vi "Eagle Scanner and Illumination Control V1.vi"() -> ()   [LabVIEW 2015]
uses:
  <vilib>/userdefined/High Color/IMAQdx.ctl
  <vilib>/vision/Image Controls.llb/IMAQ Image.ctl
  IP Dev Area/IP results.ctl
  <vilib>/FPGAPlugInAG/cRIO-9030/niLvFpga_Open_cRIO-9030.vi
  <vilib>/rvi/interface/common/dynamic/niFpgaDynamicAddResources.vi
  <vilib>/FPGAPlugInAG/Dynamic/niLvFpga_Download_Dynamic.vi
  <vilib>/FPGAPlugInAG/Dynamic/niLvFpga_Run_Dynamic.vi
  <vilib>/Utility/error.llb/Error Cluster From Error Code.vi
  <vilib>/rvi/errors/niLvFpgaAdjustHostInterfaceError.vi
  <vilib>/rvi/interface/nirviOpenFPGA/nirviOpenFPGA.xnode
  FPGA Bitfiles/BELKINEAGLEGUI_FPGATarget_EagleFPGAScanner_lK+EHUuZRCQ.lvbitx
  <vilib>/rvi/interface/nirviMethod/nirviMethod.xnode
  <vilib>/rvi/interface/nirviReadWriteControl/nirviReadWriteControl.xnode
  <vilib>/rvi/interface/Simulation/niFpgaSimulationCallBeginRW.vi
  NiFpgaLv.dll
  <vilib>/Utility/miscctls.llb/LVRectTypeDef.ctl
  <vilib>/vision/driver/NI_Vision_Acquisition_Software.lvlib
  <vilib>/vision/NI_Vision_Development_Module.lvlib
panel:
  out "LiveImageBuffer":T1
  in  "LiveVideo":bool
  out "ImagesFolder":path
  out "ImageBuffer":T1
  out "IMAQ Session":T2 caption="Session Out"
  in  "Auto Scanner":bool
  out "Tab Control":T3(tab)
  in  "Images Root Folder":path
  in  "LED Ctrl":dbl(slide)=1.0 caption="LED Ring" max=100.0 step=1.0 scale=0.0..100.0 scale format="%#.3g"
  in  "Red Dots Ctrl":dbl(slide)=1.0 caption="Red Dots" max=100.0 step=1.0 scale=0.0..100.0 scale format="%#.3g"
  in  "Number Of Points AC":u16=100 caption="Number Of Points"
  in  "Dwell Time":dbl=1.0 caption="Dwell Time [Sec]"
  in  "Radius A AC":dbl caption="Radius A [Volt]"
  in  "Radius B AC":dbl caption="Radius B [Volt]"
  in  "VY OFFS [Volt] AC":fxp<+/-,20,5> caption="VY OFFS [Volt]"
  in  "VX OFFS [Volt] AC":fxp<+/-,20,5> caption="VX OFFS [Volt]"
  out "Image":T1(plugin-control)
  in  "Run":bool
  in  "Stop":bool
  in  "A ON":bool caption="On/Off"
  in  "H ON":bool caption="On/Off"
  in  "V ON":bool caption="On/Off"
  in  "Aiming Ctrl":dbl=1.0 caption="Aiming" max=100.0 step=1.0
  in  "H Range Ctrl":dbl=1.0 caption="H Range" max=100.0 step=1.0
  in  "V Range Ctrl":dbl=1.0 caption="V Range" max=100.0 step=1.0
  in  "Scanner X":dbl=6.712328767123287 caption="X Control" min=-10.0 max=10.0 step=1.0
  in  "Scanner Y":dbl=1.5068493150684925 caption="Y Control" min=-10.0 max=10.0 step=1.0
  out "X IND":fxp<+/-,20,5>
  out "Y IND":fxp<+/-,20,5>
  in  "Send":bool
  out "X Readback Man":fxp<+/-,20,5> caption="X Readback [Volt]"
  out "Y Readback Man":fxp<+/-,20,5> caption="Y Readback [Volt]"
  out "Sensor 1":dbl
  out "Sensor 2":dbl
  out "Live Image":T1(plugin-control)
  in  "Grab":bool
  out "X Graph":u16[](graph) caption="Brightness Distribution [X]"
  out "Y Graph":u16[](graph) caption="Brightness Distribution [Y]"
  in  "AutoPlot":bool caption="Mark this to show distribution\nof the brightest point"
  in  "Snap":bool
  in  "Save":bool
  out "Y Readback":fxp<+/-,20,5> caption="Y Readback [Volt]"
  out "X Readback":fxp<+/-,20,5> caption="X Readback [Volt]"
  out "Y Command":fxp<+/-,20,5> caption="Y Command [Volt]"
  out "X Command":fxp<+/-,20,5> caption="X Command [Volt}"
  in  "Radius B":dbl caption="Radius B [Volt]"
  in  "Radius A":dbl caption="Radius A [Volt]"
  in  "Velocity":dbl=1.0 caption="Velocity [R/Sec]"
  in  "Number Of Points":u16=100
  in  "FreeRun":bool
  in  "VX OFFS [Volt]":fxp<+/-,20,5>
  in  "VY OFFS [Volt]":fxp<+/-,20,5>
  in  "Scanner FreeRun":bool
  in  "Manual Scanner":bool
  out "Stopped":bool
  in  "stop":bool
  # "EAGLE SYSTEM BASIC CONTROL"
  # "Automatic Scanner Control"
  # "Live Video"
  # "Manual Control"
  # "Illumination Control"
  # "Camera Control"
  # "Scanner Control"
  # "Otherwise touch the image at the point of interest"
  # "Temperature Sensors"
  # "Scanner Free Run"
  # "General Parameters"
  # "Calibration Parameters"
  # "Position Indication"
  # "Trajectory Parameters"
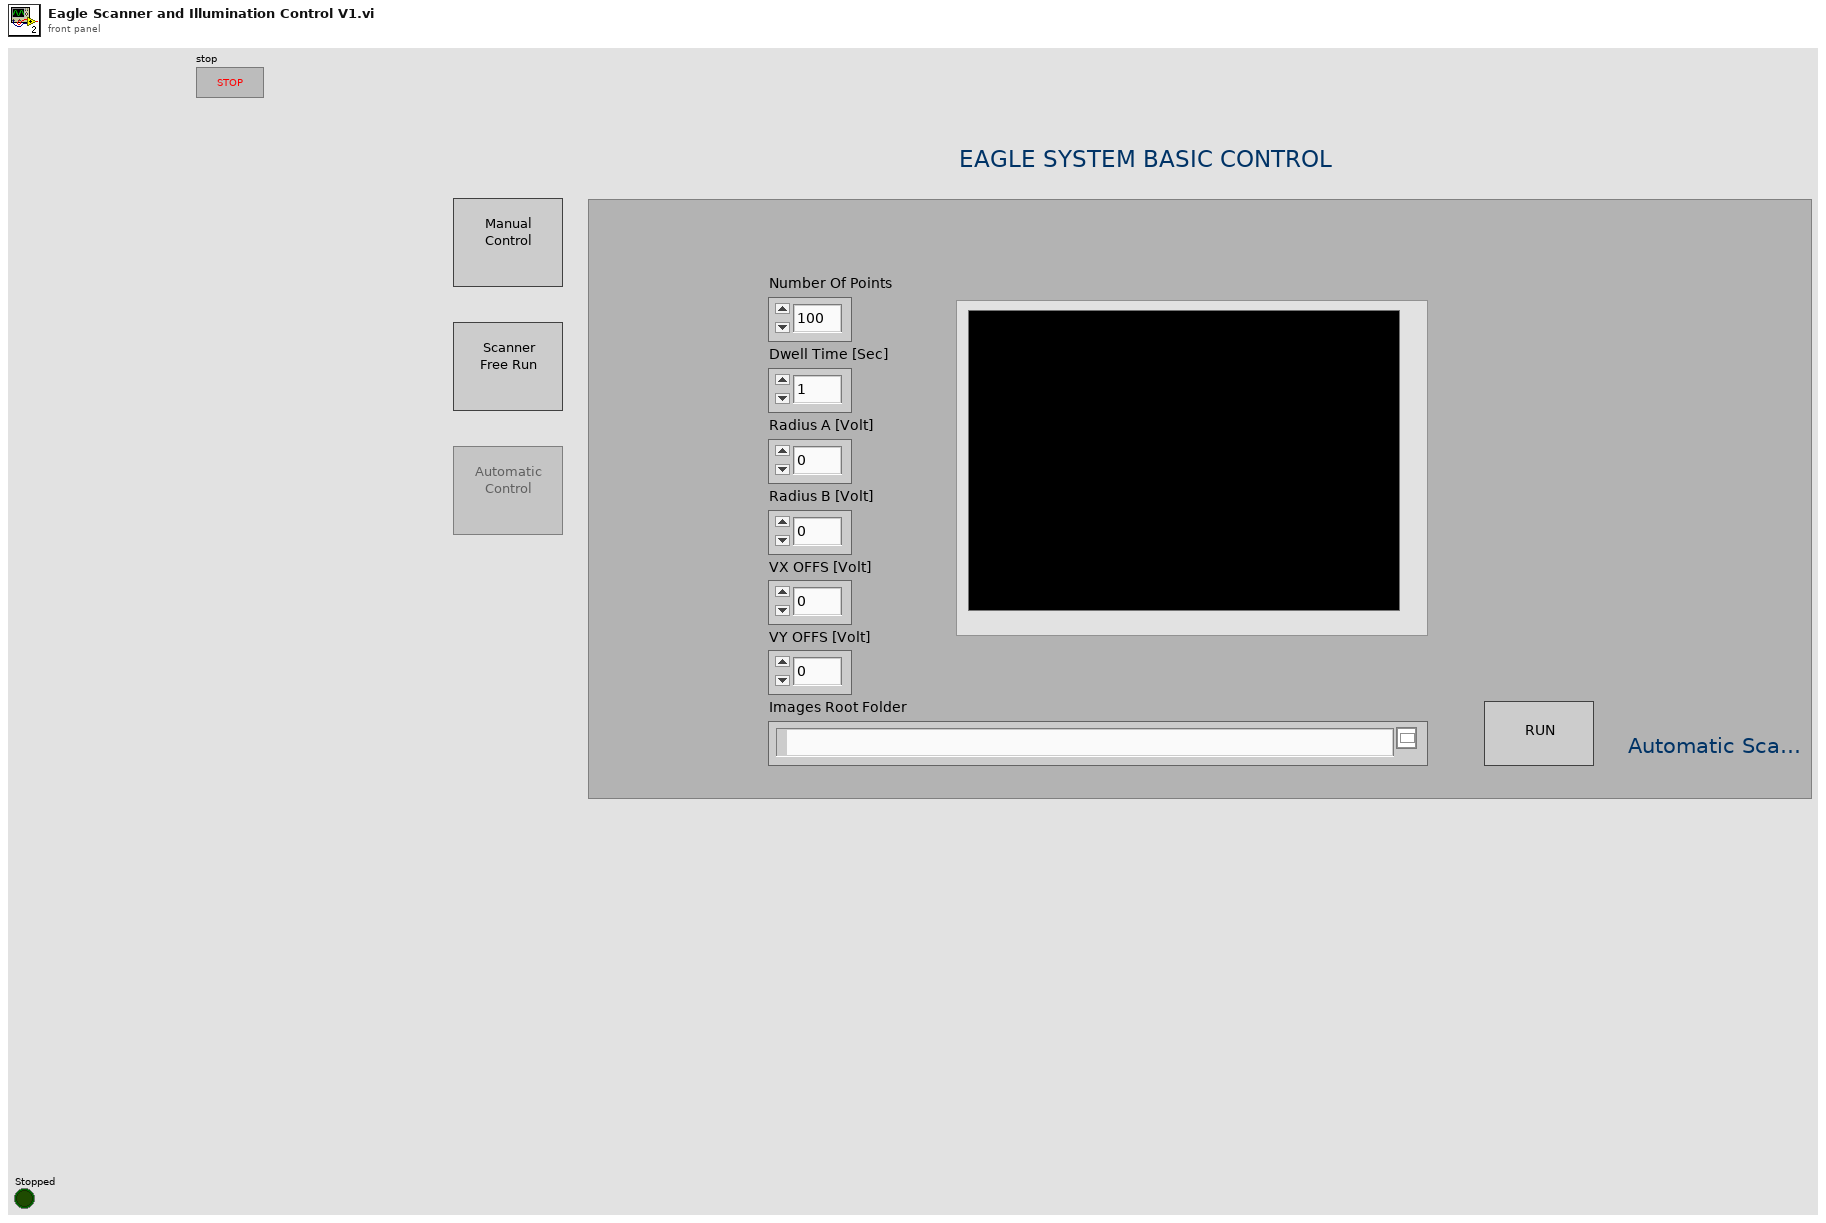
[diagram p1: front panel]
types:
  T1 = typedef "IMAQ Image.ctl" = refnum<image>
  T2 = typedef "IMAQdx.ctl" = refnum<k21>
  T3 = enum32{"Automatic", "Video Live", "Manual", "Free Run"}
  T4 = typedef "LVRectTypeDef.ctl" = cluster{"Left":i16, "Top":i16, "Right":i16, "Bottom":i16}
  T5 = cluster{"LedRing_Ctrl":dbl, "RedDots_Ctrl":dbl, "VRange_Ctrl":dbl, "HRange_Ctrl":dbl, "Aim_Ctrl":dbl, "ScanX":dbl, "ScanY":dbl, "Trajectory":cluster{"Radius A":dbl, "Radius B":dbl, "VX OFFS":fxp<+/-,20,5>, "VY OFFS":fxp<+/-,20,5>}, "General":cluster{"NumOfPoints":u16, "Velocity":dbl}, "Tab":u32, "Automatic":cluster{"NumOfPoints":u16, "Dwell Time":dbl, "VY OFFS":fxp<+/-,20,5>, "VX OFFS":fxp<+/-,20,5>, "Radius A":dbl, "Radius B":dbl}, "Images Folder":path}
  T6 = typedef "IP results.ctl" = cluster{"X":u16, "Y":u16, "A":dbl, "B":dbl, "Grade":u16, "Frame#":u16}
  T7 = enum8{"Enabled", "Disabled", "Disabled and Grayed Out"}
  T8 = typedef "Image Type" = u32
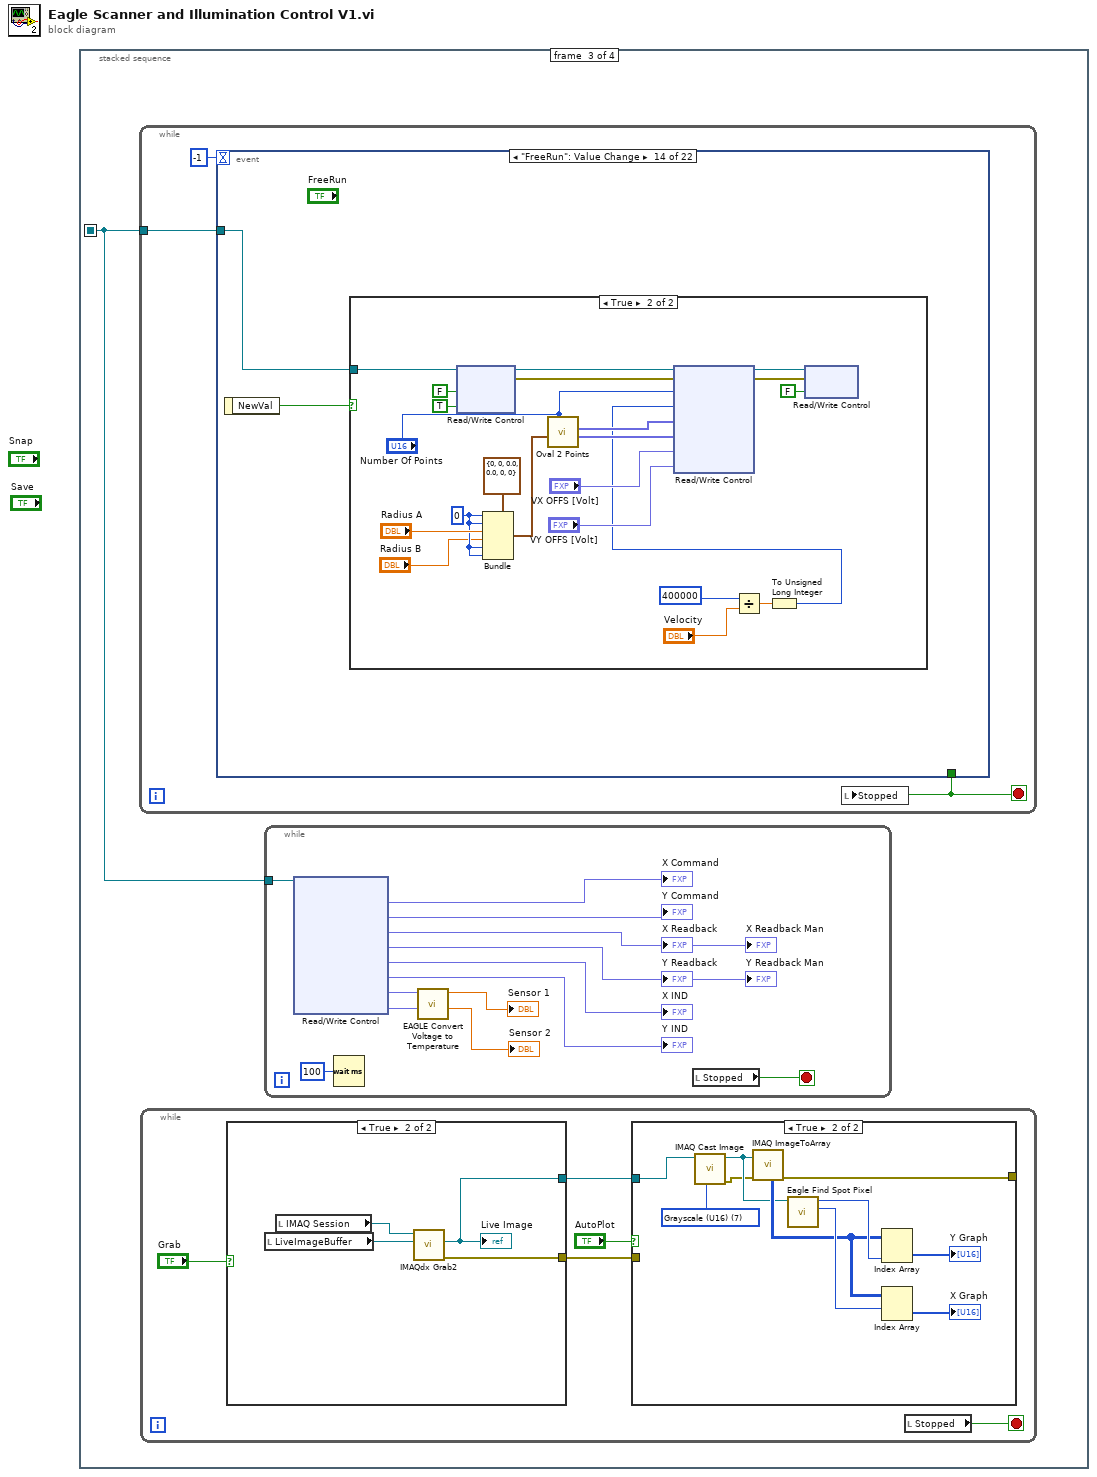
[diagram p0: block diagram]
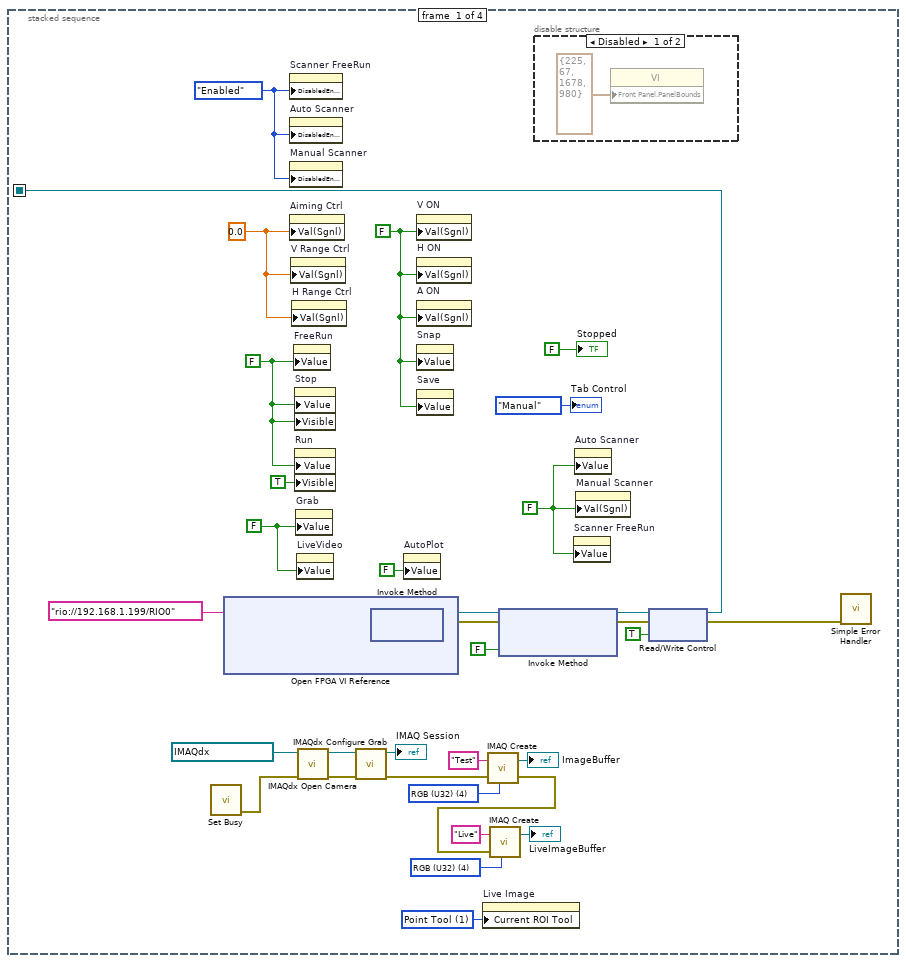
[diagram p2: hidden frame]
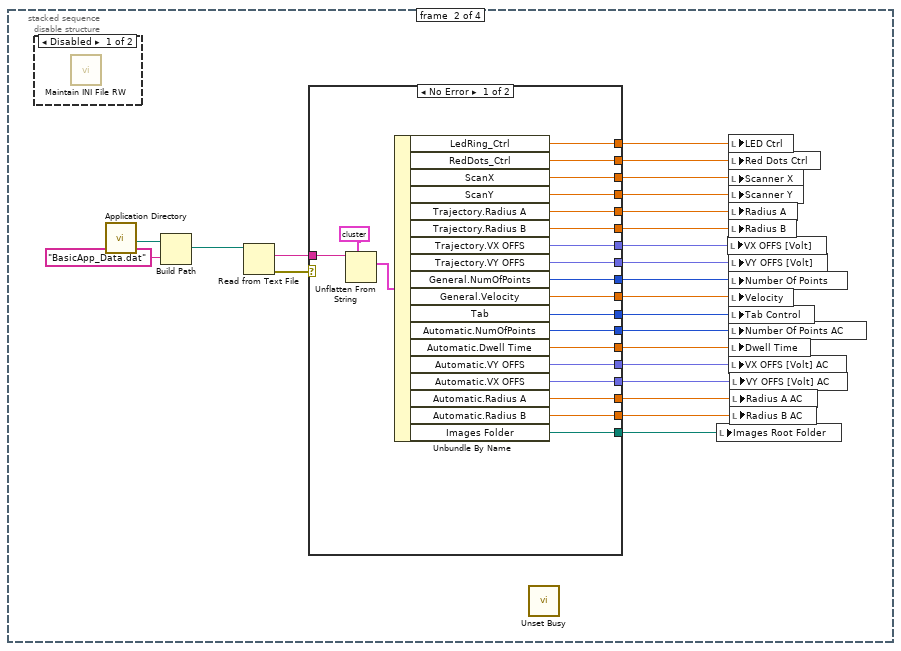
[diagram p4: hidden frame]
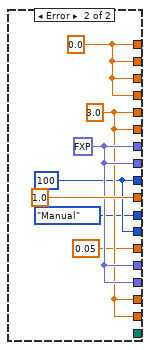
[diagram p6: hidden frame]
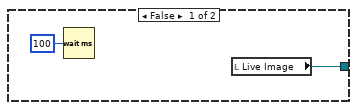
[diagram p8: hidden frame]
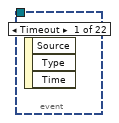
[diagram p9: hidden frame]
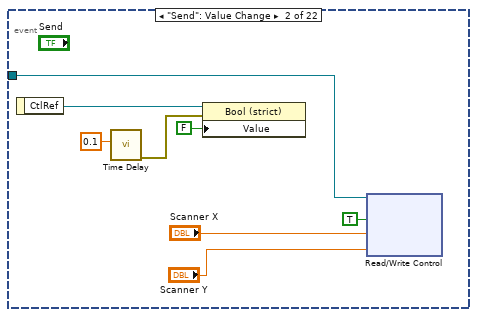
[diagram p10: hidden frame]
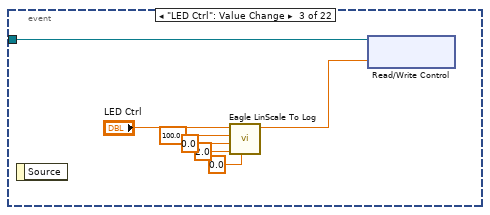
[diagram p11: hidden frame]
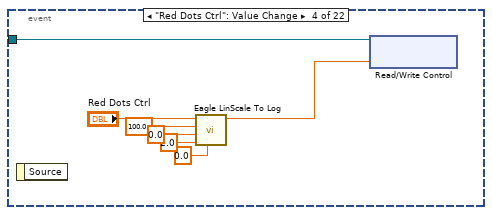
[diagram p12: hidden frame]
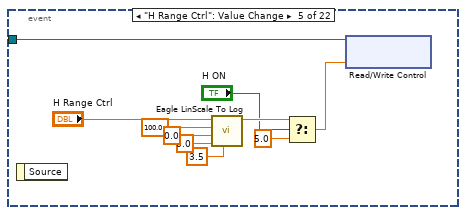
[diagram p13: hidden frame]
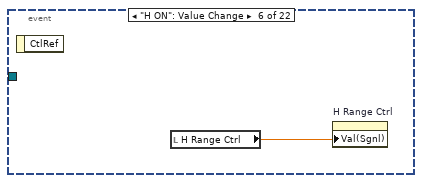
[diagram p14: hidden frame]
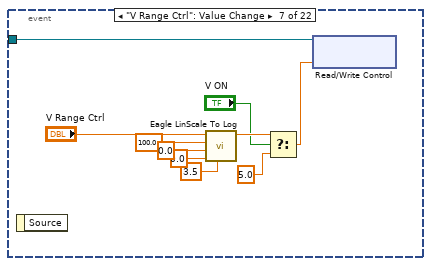
[diagram p15: hidden frame]
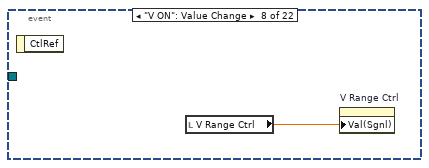
[diagram p16: hidden frame]
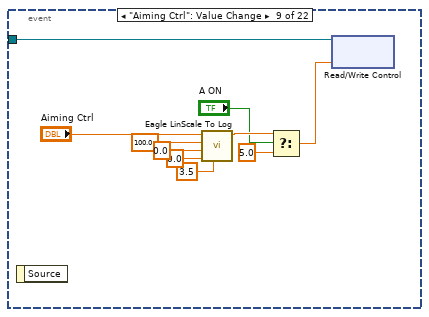
[diagram p17: hidden frame]
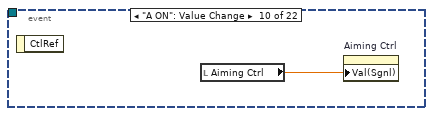
[diagram p18: hidden frame]
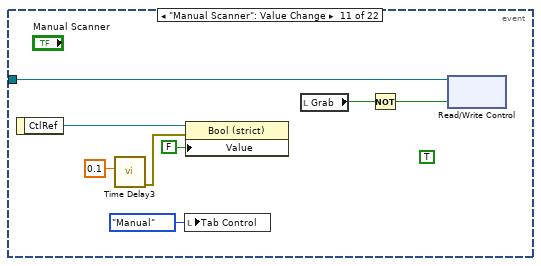
[diagram p19: hidden frame]
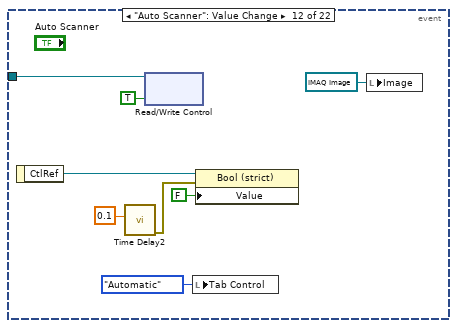
[diagram p20: hidden frame]
diagram:
  n1 = stacked-sequence {
    seq-local: [w33 _ _ _] -> [_ _ w88 _]
    frame #0 {
      w1 = FALSE
      w2 = u32 1 items=["Zoom Tool"=8, "Selection Tool"=0, "Pan Tool"=9, "Point Tool"=1, "Line Tool"=2, "Rectangle Tool"=3, "Rotated Rectangle Tool"=12, "Polyline Tool"=10, "Polygon Tool"=5, "Freehand Tool"=11, "Closed Freehand Tool"=6, "Ellipse Tool"=4, "Annulus Tool"=7] ("Current ROI Tool")
      w5 = T8 4 items=["Grayscale (U8)", "Grayscale (I16)", "Grayscale (SGL)", "Complex (CSG)", "RGB (U32)", "HSL (U32)", "RGB (U64)", "Grayscale (U16)"] ("Image Type")
      w8 = T8 4 items=["Grayscale (U8)", "Grayscale (I16)", "Grayscale (SGL)", "Complex (CSG)", "RGB (U32)", "HSL (U32)", "RGB (U64)", "Grayscale (U16)"] ("Image Type")
      w18 = FALSE ("Start Live")
      w20 = T7."Enabled" ("Disabled")
      w22 = FALSE ("FreeRun")
      w24 = 0.0 ("Value (Signaling)")
      w23 = FALSE
      n2 = call <vilib>:"Set Busy.vi"() -> ("error out"=w6:errorcluster)  [unwired: 10 in, 1 out]
      n3 = xnode "Open FPGA VI Reference"("resource name"=tag "rio://192.168.1.199/RIO0") -> ("FPGA VI Reference Out"=w30:refnum<k20>, "error out"=w29:errorcluster)  [unwired: 1 in]
      n4 = property on="Scanner FreeRun" class="Bool (strict)"("DisabledEnum"=w20) -> ()  [unwired: 2 in, 2 out]
      n5 = property on="Auto Scanner" class="Bool (strict)"("DisabledEnum"=w20) -> ()  [unwired: 2 in, 2 out]
      n6 = property on="Manual Scanner" class="Bool (strict)"("DisabledEnum"=w20) -> ()  [unwired: 2 in, 2 out]
      n7 = property on="Aiming Ctrl" class="DigNum (strict)"("Val(Sgnl)"=w24) -> ()  [unwired: 2 in, 2 out]
      n8 = property on="V Range Ctrl" class="DigNum (strict)"("Val(Sgnl)"=w24) -> ()  [unwired: 2 in, 2 out]
      n9 = property on="H Range Ctrl" class="DigNum (strict)"("Val(Sgnl)"=w24) -> ()  [unwired: 2 in, 2 out]
      n10 = property on="FreeRun" class="Bool (strict)"("Value"=w22) -> ()  [unwired: 2 in, 2 out]
      n11 = property on="Stop" class="Bool (strict)"("Value"=w22, "Visible"=w22) -> ()  [unwired: 2 in, 2 out]
      n12 = property on="Run" class="Bool (strict)"("Value"=w22, "Visible"=TRUE) -> ()  [unwired: 2 in, 2 out]
      n13 = property on="Grab" class="Bool (strict)"("Value"=w18) -> ()  [unwired: 2 in, 2 out]
      n14 = property on="LiveVideo" class="Bool (strict)"("Value"=w18) -> ()  [unwired: 2 in, 2 out]
      n15 = call <vilib>:"IMAQdx Open Camera.vi"("error in"=w6, "Session In"=T2 "acA800-200gc") -> ("error out"=w13:errorcluster, "Session Out"=w11:T2)  [unwired: 8 in]
      n16 = call <vilib>:"IMAQdx Configure Grab.vi"("error in"=w13, "Session In"=w11) -> ("error out"=w14:errorcluster, "Session Out"=→"IMAQ Session":T2)  [unwired: 8 in]
      n17 = xnode "Invoke Method"("FPGA VI Reference In"=w30, "error in"=w29) -> ("FPGA VI Reference Out"=w28:refnum<k20>, "error out"=w27:errorcluster)
      n18 = property on="AutoPlot" class="Bool (strict)"("Value"=FALSE ("AutoPlot")) -> ()  [unwired: 2 in, 2 out]
      n19 = property on="V ON" class="Bool (strict)"("Val(Sgnl)"=w1) -> ()  [unwired: 2 in, 2 out]
      n20 = property on="H ON" class="Bool (strict)"("Val(Sgnl)"=w1) -> ()  [unwired: 2 in, 2 out]
      n21 = property on="A ON" class="Bool (strict)"("Val(Sgnl)"=w1) -> ()  [unwired: 2 in, 2 out]
      n22 = property on="Snap" class="Bool (strict)"("Value"=w1) -> ()  [unwired: 2 in, 2 out]
      n23 = property on="Save" class="Bool (strict)"("Value"=w1) -> ()  [unwired: 2 in, 2 out]
      n24 = property on="Live Image" class="ImageControl"("Current ROI Tool"=w2) -> ()  [unwired: 2 in, 2 out]
      n25 = call "IMAQ Create"("Image Name"="Test", "Image Type"=w8, "error in (no error)"=w14) -> ("New Image"=→"ImageBuffer":T1, "error out"=w7:errorcluster)  [unwired: 2 in]
      n26 = call "IMAQ Create"("Image Name"="Live", "Image Type"=w5, "error in (no error)"=w7) -> ("New Image"=→"LiveImageBuffer":T1)  [unwired: 2 in, 1 out]
      n27 = xnode "Invoke Method"("FPGA VI Reference In"=w28, "error in"=w27, "Wait Until Done (F)"=FALSE) -> ("FPGA VI Reference Out"=w26:refnum<k20>, "error out"=w25:errorcluster)
      n28 = disable-structure shown="Disabled" {
        frame Disabled {
          n29 = property class="VI"("Front Panel.PanelBounds"=T4 {"Left"=225, "Top"=67, "Right"=1678, "Bottom"=980} ("Front Panel Window:Panel Bounds")) -> ()  [unwired: 2 in, 2 out]
        }
        frame Enabled {
        }
      }
      n30 = property on="Scanner FreeRun" class="Bool (strict)"("Value"=w23) -> ()  [unwired: 2 in, 2 out]
      n31 = property on="Auto Scanner" class="Bool (strict)"("Value"=w23) -> ()  [unwired: 2 in, 2 out]
      n32 = property on="Manual Scanner" class="Bool (strict)"("Val(Sgnl)"=w23) -> ()  [unwired: 2 in, 2 out]
      n33 = xnode "Read/Write Control"("FPGA VI Reference In"=w26, "error in"=w25, "Manual"=TRUE) -> ("FPGA VI Reference Out"=w33:refnum<k20>, "error out"=w31:errorcluster)
      n34 = call <vilib>:"Simple Error Handler.vi"("error in (no error)"=w31) -> ()  [unwired: 4 in, 5 out]
      "Stopped" <- FALSE ("Stopped")
      "Tab Control" <- T3."Manual" ("Tab Control")
    }
    frame #1 {
      n35 = disable-structure shown="Disabled" {
        frame Disabled {
          n36 = call "Maintain INI File RW.vi"() -> ()  [unwired: 11 in, 1 out]
        }
        frame Enabled {
        }
      }
      n37 = call <vilib>:"Application Directory.vi"() -> ("Application Directory"=w59:path)
      n38 = Build Path(base path=w59, name or relative path="BasicApp_Data.dat") -> (appended path=w57:path)
      n39 = Read from Text File(file (use dialog)=w57) -> (text=w55:string, error out=w56:errorcluster)  [unwired: 3 in, 2 out]
      n40 = case shown="No Error" w56 {
        tunnel: w55 -> [w80 _]
        tunnel: [w78 w87] -> w54
        tunnel: [w77 w87] -> w53
        tunnel: [w76 w87] -> w52
        tunnel: [w75 w87] -> w51
        tunnel: [w74 w84] -> w50
        tunnel: [w73 w84] -> w49
        tunnel: [w72 w82] -> w48
        tunnel: [w71 1.0 ("Velocity")] -> w47
        tunnel: [w70 T3."Manual" ("Tab Control")] -> w37
        tunnel: [w69 w85] -> w46
        tunnel: [w68 w85] -> w45
        tunnel: [w67 w82] -> w39
        tunnel: [w66 0.05 ("Dwell Time")] -> w40
        tunnel: [w65 w85] -> w41
        tunnel: [w64 w85] -> w42
        tunnel: [w63 w84] -> w43
        tunnel: [w62 w84] -> w44
        tunnel: [w60 _] -> w38
        frame No Error {
          n41 = Unflatten From String(type=T5 {"LedRing_Ctrl"=0.0, "RedDots_Ctrl"=0.0, "VRange_Ctrl"=0.0, "HRange_Ctrl"=0.0, "Aim_Ctrl"=0.0, "ScanX"=0.0, "ScanY"=0.0, "Trajectory"={"Radius A"=0.0, "Radius B"=0.0, "VX OFFS"=0.0, "VY OFFS"=0.0}, "General"={"NumOfPoints"=0, "Velocity"=0.0}, "Tab"=0, "Automatic"={"NumOfPoints"=0, "Dwell Time"=0.0, "VY OFFS"=0.0, "VX OFFS"=0.0, "Radius A"=0.0, "Radius B"=0.0}, "Images Folder"=path ""} ("PanelData"), binary string=w80) -> (value=w79:T5)  [unwired: 3 in, 2 out]
          n42 = Unbundle By Name(w79) -> ("LedRing_Ctrl"=w78:dbl, "RedDots_Ctrl"=w77:dbl, "ScanX"=w76:dbl, "ScanY"=w75:dbl, "Trajectory.Radius A"=w74:dbl, "Trajectory.Radius B"=w73:dbl, "Trajectory.VX OFFS"=w69:fxp<+/-,20,5>, "Trajectory.VY OFFS"=w68:fxp<+/-,20,5>, "General.NumOfPoints"=w72:u16, "General.Velocity"=w71:dbl, "Tab"=w70:u32, "Automatic.NumOfPoints"=w67:u16, "Automatic.Dwell Time"=w66:dbl, "Automatic.VY OFFS"=w65:fxp<+/-,20,5>, "Automatic.VX OFFS"=w64:fxp<+/-,20,5>, "Automatic.Radius A"=w63:dbl, "Automatic.Radius B"=w62:dbl, "Images Folder"=w60:path)
        }
        frame Error {
          w85 = fxp<+/-,20,5> 0.0 ("VX OFFS")
          w84 = 3.0 ("Radius A")
          w82 = u16 100 ("NumOfPoints")
          w87 = 0.0 ("LedRing_Ctrl")
        }
      }
      n43 = call <vilib>:"Unset Busy.vi"() -> ()  [unwired: 11 in, 1 out]
      n44 = local write "Images Root Folder"(w38) -> ()
      n45 = local write "VX OFFS [Volt]"(w46) -> ()
      n46 = local write "LED Ctrl"(w54) -> ()
      n47 = local write "Red Dots Ctrl"(w53) -> ()
      n48 = local write "Scanner X"(w52) -> ()
      n49 = local write "Scanner Y"(w51) -> ()
      n50 = local write "Radius A"(w50) -> ()
      n51 = local write "Radius B"(w49) -> ()
      n52 = local write "VY OFFS [Volt]"(w45) -> ()
      n53 = local write "Number Of Points"(w48) -> ()
      n54 = local write "Velocity"(w47) -> ()
      n55 = local write "Tab Control"(w37) -> ()
      n56 = local write "Number Of Points AC"(w39) -> ()
      n57 = local write "Dwell Time"(w40) -> ()
      n58 = local write "VX OFFS [Volt] AC"(w41) -> ()
      n59 = local write "VY OFFS [Volt] AC"(w42) -> ()
      n60 = local write "Radius A AC"(w43) -> ()
      n61 = local write "Radius B AC"(w44) -> ()
    }
    frame #2 {
      n62 = while {
        tunnel: w88 -> [w125]
        stop <- w124 stop-if-true
        n63 = event shown="[13] \"FreeRun\": Value Change" {
          selector: _ -> [_ _ _ _ _ _ _ _ _ _ _ _ _ _ _ _ _ _ _ _ _ _]
          dyn-events: _ -> [_ _ _ _ _ _ _ _ _ _ _ _ _ _ _ _ _ _ _ _ _ _]
          timeout: -1 -> [_ _ _ _ _ _ _ _ _ _ _ _ _ _ _ _ _ _ _ _ _ _]
          tunnel: [_ _ _ _ _ _ _ _ _ _ _ _ _ _ _ _ w329 _ _ _ _ _] -> w124
          tunnel: w125 -> [_ w129 w140 w147 w157 _ w168 _ w179 _ w184 w191 w201 w207 _ w238 _ _ _ _ _ _]
          event Timeout {
            n64 = event-data() -> ()  [unwired: 1 in, 3 out]
          }
          event "Send": Value Change {
            n65 = event-data() -> ("CtlRef"=w133:refnum<vi>)  [unwired: 1 in]
            n66 = call "Time Delay"("Delay Time (s)"=0.1) -> ("error out"=w131:errorcluster)  [unwired: 10 in]
            n67 = property class="Bool (strict)"(reference=w133, error in=w131, "Value"=FALSE) -> ()  [unwired: 2 out]
            n68 = xnode "Read/Write Control"("FPGA VI Reference In"=w129, "Manual"=TRUE, "Manual VX"="Scanner X", "Manual VY"="Scanner Y") -> ()  [unwired: 1 in, 2 out]
          }
          event "LED Ctrl": Value Change {
            n69 = event-data() -> ()  [unwired: 1 in, 1 out]
            n70 = call "Eagle LinScale To Log.vi"("MinScaleOut"=0.0, "MaxScaleOut"=2.0, "MinScaleIn"=0.0, "MaxScaleIn"=100.0, "ValIn"="LED Ctrl") -> ("ValOut"=w134:dbl)  [unwired: 6 in]
            n71 = xnode "Read/Write Control"("FPGA VI Reference In"=w140, "LED Ring Ctrl"=w134) -> ()  [unwired: 1 in, 2 out]
          }
          event "Red Dots Ctrl": Value Change {
            n72 = event-data() -> ()  [unwired: 1 in, 1 out]
            n73 = call "Eagle LinScale To Log.vi"("MinScaleOut"=0.0, "MaxScaleOut"=2.0, "MinScaleIn"=0.0, "MaxScaleIn"=100.0, "ValIn"="Red Dots Ctrl") -> ("ValOut"=w141:dbl)  [unwired: 6 in]
            n74 = xnode "Read/Write Control"("FPGA VI Reference In"=w147, "Red Dots Ctrl"=w141) -> ()  [unwired: 1 in, 2 out]
          }
          event "H Range Ctrl": Value Change {
            n75 = event-data() -> ()  [unwired: 1 in, 1 out]
            n76 = call "Eagle LinScale To Log.vi"("MinScaleOut"=3.5, "MaxScaleOut"=0.0, "MinScaleIn"=0.0, "MaxScaleIn"=100.0, "ValIn"="H Range Ctrl") -> ("ValOut"=w151:dbl)  [unwired: 6 in]
            n77 = Select(t=w151, s="H ON", f=5.0) -> (s? t:f=w148:dbl)
            n78 = xnode "Read/Write Control"("FPGA VI Reference In"=w157, "H Range Ctrl"=w148) -> ()  [unwired: 1 in, 2 out]
          }
          event "H ON": Value Change {
            n79 = event-data() -> ()  [unwired: 1 in, 1 out]
            n80 = local read "H Range Ctrl"() -> (w158:dbl)
            n81 = property on="H Range Ctrl" class="DigNum (strict)"("Val(Sgnl)"=w158) -> ()  [unwired: 2 in, 2 out]
          }
          event "V Range Ctrl": Value Change {
            n82 = event-data() -> ()  [unwired: 1 in, 1 out]
            n83 = call "Eagle LinScale To Log.vi"("MinScaleOut"=3.5, "MaxScaleOut"=0.0, "MinScaleIn"=0.0, "MaxScaleIn"=100.0, "ValIn"="V Range Ctrl") -> ("ValOut"=w162:dbl)  [unwired: 6 in]
            n84 = Select(t=w162, s="V ON", f=5.0) -> (s? t:f=w161:dbl)
            n85 = xnode "Read/Write Control"("FPGA VI Reference In"=w168, "V Range Ctrl"=w161) -> ()  [unwired: 1 in, 2 out]
          }
          event "V ON": Value Change {
            n86 = event-data() -> ()  [unwired: 1 in, 1 out]
            n87 = local read "V Range Ctrl"() -> (w169:dbl)
            n88 = property on="V Range Ctrl" class="DigNum (strict)"("Val(Sgnl)"=w169) -> ()  [unwired: 2 in, 2 out]
          }
          event "Aiming Ctrl": Value Change {
            n89 = event-data() -> ()  [unwired: 1 in, 1 out]
            n90 = call "Eagle LinScale To Log.vi"("MinScaleOut"=3.5, "MaxScaleOut"=0.0, "MinScaleIn"=0.0, "MaxScaleIn"=100.0, "ValIn"="Aiming Ctrl") -> ("ValOut"=w173:dbl)  [unwired: 6 in]
            n91 = Select(t=w173, s="A ON", f=5.0) -> (s? t:f=w170:dbl)
            n92 = xnode "Read/Write Control"("FPGA VI Reference In"=w179, "Aim Ctrl"=w170) -> ()  [unwired: 1 in, 2 out]
          }
          event "A ON": Value Change {
            n93 = event-data() -> ()  [unwired: 1 in, 1 out]
            n94 = local read "Aiming Ctrl"() -> (w180:dbl)
            n95 = property on="Aiming Ctrl" class="DigNum (strict)"("Val(Sgnl)"=w180) -> ()  [unwired: 2 in, 2 out]
          }
          event "Manual Scanner": Value Change {
            (unwired) TRUE ("Manual")
            n96 = event-data() -> ("CtlRef"=w185:refnum<vi>)  [unwired: 1 in]
            n97 = call "Time Delay3"("Delay Time (s)"=0.1) -> ("error out"=w187:errorcluster)  [unwired: 10 in]
            n98 = local write "Tab Control"(T3."Manual" ("Tab Control")) -> ()
            n99 = property class="Bool (strict)"(reference=w185, error in=w187, "Value"=FALSE) -> ()  [unwired: 2 out]
            n100 = local read "Grab"() -> (w182:bool)
            n101 = Not(x=w182) -> (.not. x?=w181:bool)
            n102 = xnode "Read/Write Control"("FPGA VI Reference In"=w184, "Manual"=w181) -> ()  [unwired: 1 in, 2 out]
          }
          event "Auto Scanner": Value Change {
            n103 = event-data() -> ("CtlRef"=w193:refnum<vi>)  [unwired: 1 in]
            n104 = call "Time Delay2"("Delay Time (s)"=0.1) -> ("error out"=w195:errorcluster)  [unwired: 10 in]
            n105 = xnode "Read/Write Control"("FPGA VI Reference In"=w191, "Manual"=TRUE) -> ()  [unwired: 1 in, 2 out]
            n106 = local write "Tab Control"(T3."Automatic" ("Tab Control")) -> ()
            n107 = property class="Bool (strict)"(reference=w193, error in=w195, "Value"=FALSE) -> ()  [unwired: 2 out]
            n108 = local write "Image"(T1 refnum ("Image")) -> ()
          }
          event "Scanner FreeRun": Value Change {
            n109 = event-data() -> ("CtlRef"=w202:refnum<vi>)  [unwired: 1 in]
            n110 = call "Time Delay4"("Delay Time (s)"=0.1) -> ("error out"=w204:errorcluster)  [unwired: 10 in]
            n111 = local write "Tab Control"(T3."Free Run" ("Tab Control")) -> ()
            n112 = property class="Bool (strict)"(reference=w202, error in=w204, "Value"=FALSE) -> ()  [unwired: 2 out]
            n113 = xnode "Read/Write Control"("FPGA VI Reference In"=w201, "Manual"=TRUE) -> ("error out"=w197:errorcluster)  [unwired: 1 in, 1 out]
            n114 = property on="FreeRun" class="Bool (strict)"(error in=w197, "Value"=FALSE ("FreeRun")) -> ()  [unwired: 1 in, 2 out]
          }
          event "FreeRun": Value Change {
            n115 = event-data() -> ("NewVal"=w206:bool)  [unwired: 1 in]
            n116 = case shown="True" w206 {
              tunnel: w207 -> [w209 w231]
              frame False {
                n117 = xnode "Read/Write Control"("FPGA VI Reference In"=w209, "Reset"=TRUE) -> ()  [unwired: 1 in, 2 out]
              }
              frame True {
                w223 = u16 0 ("X")
                n118 = xnode "Read/Write Control"("FPGA VI Reference In"=w231, "Manual"=FALSE ("Reset"), "Reset"=TRUE) -> ("FPGA VI Reference Out"=w229:refnum<k20>, "error out"=w215:errorcluster)  [unwired: 1 in]
                n119 = Bundle(cluster=T6 {"X"=0, "Y"=0, "A"=0.0, "B"=0.0, "Grade"=0, "Frame#"=0} ("IP Results"), "X"=w223, "Y"=w223, "A"="Radius A", "B"="Radius B", "Grade"=w223, "Frame#"=w223) -> (w225:T6)
                n120 = call "Oval 2 Points .vi"("NoOfPoints"="Number Of Points", "IP Results"=w225) -> ("Y Points"=w227:fxp<+/-,20,5>[], "X Points"=w228:fxp<+/-,20,5>[])  [unwired: 8 in]
                n121 = Divide(x=400000, y="Velocity") -> (x/y=w211:dbl)
                n122 = To Unsigned Long Integer(number=w211) -> (unsigned 32bit integer=w210:u32)
                n123 = xnode "Read/Write Control"("FPGA VI Reference In"=w229, "error in"=w215, "NoOfPoints"="Number Of Points", "ScanRate"=w210, "X Array"=w228, "Y Array"=w227, "VX OFFS"="VX OFFS [Volt]", "VY OFFS"="VY OFFS [Volt]") -> ("FPGA VI Reference Out"=w217:refnum<k20>, "error out"=w216:errorcluster)
                n124 = xnode "Read/Write Control"("FPGA VI Reference In"=w217, "error in"=w216, "Reset"=FALSE) -> ()  [unwired: 2 out]
              }
            }
          }
          event "LiveVideo": Value Change {
            n125 = event-data() -> ("CtlRef"=w234:refnum<vi>)  [unwired: 1 in]
            n126 = call "Time Delay7"("Delay Time (s)"=0.1) -> ("error out"=w236:errorcluster)  [unwired: 10 in]
            n127 = local write "Tab Control"(T3."Video Live" ("Tab Control")) -> ()
            n128 = property class="Bool (strict)"(reference=w234, error in=w236, "Value"=FALSE) -> ()  [unwired: 2 out]
            n129 = local write "Live Image"(T1 refnum ("Live Image")) -> ()
          }
          event "Run": Value Change {
            n130 = event-data() -> ("CtlRef"=w239:refnum<vi>)  [unwired: 1 in]
            n131 = stacked-sequence {
              seq-local: [w256 _ _] -> [_ w275 _]
              seq-local: [w255 _ _] -> [_ w274 _]
              seq-local: [_ w271 _] -> [_ _ w322]
              tunnel: w238 -> [w264 w273 _]
              frame #0 {
                w261 = u16 0 ("X")
                w243 = T7."Disabled and Grayed Out" ("Disabled")
                w265 = FALSE ("Stop")
                n132 = Format Date/Time String(time format string (%c)="%d%m%y_%H%M%S") -> (date/time string=w250:string)  [unwired: 2 in]
                n133 = xnode "Read/Write Control"("FPGA VI Reference In"=w264, "Manual"=TRUE) -> ()  [unwired: 1 in, 2 out]
                n134 = property on="Scanner FreeRun" class="Bool (strict)"("DisabledEnum"=w243) -> ()  [unwired: 2 in, 2 out]
                n135 = property on="Auto Scanner" class="Bool (strict)"("DisabledEnum"=w243) -> ()  [unwired: 2 in, 2 out]
                n136 = property on="Manual Scanner" class="Bool (strict)"("DisabledEnum"=w243) -> ()  [unwired: 2 in, 2 out]
                n137 = property on="LiveVideo" class="Bool (strict)"("DisabledEnum"=w243) -> ()  [unwired: 2 in, 2 out]
                n138 = property on="Stop" class="Bool (strict)"("Value"=w265, "Visible"=TRUE) -> ()  [unwired: 2 in, 2 out]
                n139 = property on="Run" class="Bool (strict)"("Value"=w265, "Visible"=w265) -> ()  [unwired: 2 in, 2 out]
                n140 = Concatenate Strings("Images", "_", w250) -> (w252:string)
                n141 = Build Path(base path="Images Root Folder", name or relative path=w252) -> (appended path=w248:path)
                n142 = call <vilib>:"Check if File or Folder Exists.vi"("path"=w248) -> ("error out"=w245:errorcluster, "file or folder exists?"=w247:bool, "dup path"=w246:path)  [unwired: 8 in]
                n143 = case shown="False" w247 {
                  tunnel: w246 -> [w269 w270]
                  tunnel: [w267 w270] -> w244
                  tunnel: w245 -> [w268 _]
                  frame False {
                    n144 = Create Folder(path (use dialog)=w269, error in=w268) -> (created path=w267:path)  [unwired: 1 in, 2 out]
                  }
                  frame True {
                  }
                }
                "ImagesFolder" <- w244
                n145 = Bundle(cluster=T6 {"X"=0, "Y"=0, "A"=0.0, "B"=0.0, "Grade"=0, "Frame#"=0} ("IP Results"), "X"=w261, "Y"=w261, "A"="Radius A AC", "B"="Radius B AC", "Grade"=w261, "Frame#"=w261) -> (w262:T6)
                n146 = call "Oval 2 Points .vi"("NoOfPoints"="Number Of Points AC", "IP Results"=w262) -> ("Y Points"=w255:fxp<+/-,20,5>[], "X Points"=w256:fxp<+/-,20,5>[])  [unwired: 8 in]
              }
              frame #1 {
                n147 = while {
                  tunnel: w275 -> [w320]
                  tunnel: w274 -> [w319]
                  tunnel: w273 -> [w314]
                  shift-right: [w288] -> w271
                  shift-left: "" -> [w289]
                  i -> [w299]
                  stop <- w306 stop-if-true
                  w284 = T8 7 items=["Grayscale (U8)", "Grayscale (I16)", "Grayscale (SGL)", "Complex (CSG)", "RGB (U32)", "HSL (U32)", "RGB (U64)", "Grayscale (U16)"] ("Image Type")
                  w281 = ","
                  n148 = Increment(x=w299) -> (x+1=w298:i32)
                  n149 = Index Array(array=w320, index=w299) -> (element=w318:fxp<+/-,20,5>)
                  n150 = Index Array(array=w319, index=w299) -> (element=w317:fxp<+/-,20,5>)
                  n151 = Number To Decimal String(number=w298) -> (decimal integer string=w297:string)  [unwired: 1 in]
                  n152 = Add(x="VX OFFS [Volt] AC", y=w318) -> (x+y=w313:fxp<+/-,21,6>)
                  n153 = Add(x=w317, y="VY OFFS [Volt] AC") -> (x+y=w312:fxp<+/-,21,6>)
                  n154 = xnode "Read/Write Control"("FPGA VI Reference In"=w314, "Manual VX"=w313, "Manual VY"=w312) -> ("error out"=w311:errorcluster)  [unwired: 1 in, 1 out]
                  n155 = local read "IMAQ Session"() -> (w304:T2)
                  n156 = local read "ImagesFolder"() -> (w301:path)
                  n157 = local read "ImageBuffer"() -> (w303:T1)
                  n158 = Concatenate Strings("Image_" ("string"), w297, ".tif" ("string")) -> (w295:string)
                  n159 = local read "Number Of Points AC"() -> (w307:u16)
                  n160 = call "Time Delay6"("error in (no error)"=w311, "Delay Time (s)"="Dwell Time") -> ("error out"=w305:errorcluster)  [unwired: 9 in]
                  n161 = Build Path(base path=w301, name or relative path=w295) -> (appended path=w294:path)
                  n162 = call <vilib>:"IMAQdx Grab2.vi"("error in"=w305, "Image In"=w303, "Session In"=w304) -> ("error out"=w302:errorcluster, "Image Out"=w293:T1)  [unwired: 5 in, 2 out]
                  "Image" <- w293
                  n163 = Decrement(x=w307) -> (x-1=w286:u16)
                  n164 = Greater Or Equal?(x=w299, y=w286) -> (x >= y?=w308:bool)
                  n165 = call-poly "IMAQ Write File 2"("error in (no error)"=w302, "File Path"=w294, "Image"=w293) -> ("Image Out (duplicate)"=w285:T1)  [unwired: 7 in, 1 out]
                  n166 = Or(x="Stop", y=w308) -> (x .or. y?=w306:bool)
                  n167 = call "IMAQ Cast Image"("Image Type"=w284, "Image Src"=w285) -> ("Image Dst Out"=w283:T1)  [unwired: 8 in, 1 out]
                  n168 = call "IMAQ ImageToArray"("Image"=w283) -> ("Image Pixels (U16)"=w282:u16[][])  [unwired: 3 in, 4 out]
                  n169 = call "Eagle Find Spot Pixel.vi"("Load From File"=FALSE, "Image"=w283) -> ("Y Pixel"=w276:i32, "X Pixel"=w277:i32)  [unwired: 7 in, 1 out]
                  n170 = Number To Decimal String(number=w277) -> (decimal integer string=w291:string)  [unwired: 1 in]
                  n171 = Number To Decimal String(number=w276) -> (decimal integer string=w290:string)  [unwired: 1 in]
                  n172 = Index Array(array=w282, index (row)=w276, index (col)=w277) -> (element=w280:u16)
                  n173 = Number To Decimal String(number=w280) -> (decimal integer string=w279:string)  [unwired: 1 in]
                  n174 = Concatenate Strings(w291, w281, w290, w281, w279, "\r") -> (w287:string)
                  n175 = Concatenate Strings(w289, w287) -> (w288:string)
                }
              }
              frame #2 {
                w321 = T7."Enabled" ("Disabled")
                w327 = FALSE ("Stop")
                n176 = property on="LiveVideo" class="Bool (strict)"("DisabledEnum"=w321) -> ()  [unwired: 2 in, 2 out]
                n177 = property on="Scanner FreeRun" class="Bool (strict)"("DisabledEnum"=w321) -> ()  [unwired: 2 in, 2 out]
                n178 = property on="Auto Scanner" class="Bool (strict)"("DisabledEnum"=w321) -> ()  [unwired: 2 in, 2 out]
                n179 = property on="Manual Scanner" class="Bool (strict)"("DisabledEnum"=w321) -> ()  [unwired: 2 in, 2 out]
                n180 = property on="Stop" class="Bool (strict)"("Value"=w327, "Visible"=w327) -> ()  [unwired: 2 in, 2 out]
                n181 = property on="Run" class="Bool (strict)"("Value"=w327, "Visible"=TRUE) -> ()  [unwired: 2 in, 2 out]
                n182 = local read "ImagesFolder"() -> (w325:path)
                n183 = Build Path(base path=w325, name or relative path="ListOfPoints.csv") -> (appended path=w323:path)
                n184 = Write to Text File(file (use dialog)=w323, text=w322) -> ()  [unwired: 2 in, 3 out]
              }
            }
            n185 = call "Time Delay5"("Delay Time (s)"=0.1) -> ("error out"=w241:errorcluster)  [unwired: 10 in]
            n186 = property class="Bool (strict)"(reference=w239, error in=w241, "Value"=FALSE) -> ()  [unwired: 2 out]
          }
          event "stop": Value Change {
            n187 = event-data() -> ("CtlRef"=w332:refnum<vi>)  [unwired: 1 in]
            n188 = property class="Bool (strict)"(reference=w332, "Value"=FALSE) -> ()  [unwired: 1 in, 2 out]
            n189 = local write "Stopped"(TRUE ("Stopped")) -> ()
            n190 = Two Button Dialog(message="Exit this application?") -> (T button?=w329:bool)  [unwired: 2 in]
          }
          event "Grab": Value Change {
            n191 = event-data() -> ("NewVal"=w336:bool)  [unwired: 1 in]
            n192 = Select(t=T7."Disabled and Grayed Out" ("Disabled"), s=w336, f=T7."Enabled") -> (s? t:f=w333:T7)
            n193 = property on="Auto Scanner" class="Bool (strict)"("DisabledEnum"=w333) -> ()  [unwired: 2 in, 2 out]
            n194 = property on="Snap" class="Bool (strict)"("DisabledEnum"=w333) -> ()  [unwired: 2 in, 2 out]
            n195 = property on="Save" class="Bool (strict)"("DisabledEnum"=w333) -> ()  [unwired: 2 in, 2 out]
          }
          event "Snap": Value Change {
            n196 = event-data() -> ("CtlRef"=w343:refnum<vi>)  [unwired: 1 in]
            n197 = call "Time Delay8"("Delay Time (s)"=0.1) -> ("error out"=w340:errorcluster)  [unwired: 10 in]
            n198 = property class="Bool (strict)"(reference=w343, error in=w340, "Value"=FALSE) -> ()  [unwired: 2 out]
            n199 = local read "LiveImageBuffer"() -> (w338:T1)
            n200 = local read "IMAQ Session"() -> (w339:T2)
            n201 = call <vilib>:"IMAQdx Grab2.vi"("Image In"=w338, "Session In"=w339) -> ("Image Out"=w337:T1)  [unwired: 6 in, 3 out]
            n202 = local write "Live Image"(w337) -> ()
          }
          event "Save": Value Change {
            n203 = event-data() -> ("CtlRef"=w348:refnum<vi>)  [unwired: 1 in]
            n204 = call "Time Delay10"("Delay Time (s)"=0.1) -> ("error out"=w349:errorcluster)  [unwired: 10 in]
            n205 = local read "Live Image"() -> (w347:T1)
            n206 = call "File Dialog"("pattern (all files)"="*.tif;*.tiff", "pattern label"="TIFF") -> ("selected path"=w346:path)  [unwired: 10 in, 3 out]
            n207 = property class="Bool (strict)"(reference=w348, error in=w349, "Value"=FALSE) -> ()  [unwired: 2 out]
            n208 = call-poly "IMAQ Write File 2"("File Path"=w346, "Image"=w347) -> ()  [unwired: 8 in, 2 out]
          }
          event "Live Image": Mouse Down? {
            n209 = event-data() -> ("CtlRef"=w353:refnum<vi>)  [unwired: 1 in]
            n210 = local read "AutoPlot"() -> (w352:bool)
            n211 = case shown="False" w352 {
              tunnel: w353 -> [w365 _]
              tunnel: [w355 _] -> _
              frame False {
                w356 = T8 7 items=["Grayscale (U8)", "Grayscale (I16)", "Grayscale (SGL)", "Complex (CSG)", "RGB (U32)", "HSL (U32)", "RGB (U64)", "Grayscale (U16)"] ("Image Type")
                n212 = local read "Live Image"() -> (w358:T1)
                n213 = property class="ImageControl"(reference=w365) -> ("Last Mouse Position"=w363:cluster{"X":i32, "Y":i32})  [unwired: 1 in, 2 out]
                n214 = call "IMAQ Cast Image"("Image Type"=w356, "Image Src"=w358) -> ("error out"=w355:errorcluster, "Image Dst Out"=w357:T1)  [unwired: 8 in]
                n215 = Unbundle By Name(w363) -> ("X"=w362:i32, "Y"=w361:i32)
                n216 = call "IMAQ ImageToArray"("Image"=w357) -> ("Image Pixels (U16)"=w364:u16[][])  [unwired: 3 in, 4 out]
                n217 = Index Array(array=w364, index (col)=w362) -> (element=w360:u16[])  [unwired: 1 in]
                n218 = Index Array(array=w364, index (row)=w361) -> (element=w359:u16[])  [unwired: 1 in]
                n219 = local write "Y Graph"(w360) -> ()
                n220 = local write "X Graph"(w359) -> ()
              }
              frame True {
              }
            }
            n221 = event-data("Discard?"=FALSE) -> ()  [unwired: 1 in, 1 out]
          }
          event Panel Close? {
            n222 = event-data() -> ()  [unwired: 1 in, 1 out]
            n223 = property on="stop" class="Bool (strict)"("Val(Sgnl)"=FALSE ("Value (Signaling)")) -> ()  [unwired: 2 in, 2 out]
            n224 = event-data("Discard?"=TRUE) -> ()  [unwired: 1 in, 1 out]
          }
        }
        n225 = local write "Stopped"(w124) -> ()
      }
      n226 = while {
        stop <- w93 stop-if-true
        n227 = case shown="True" "Grab" {
          tunnel: [_ w109] -> w90
          tunnel: [w104 w108] -> w89
          frame False {
            n228 = Wait (ms)(milliseconds to wait=u32 100) -> ()  [unwired: 1 out]
            n229 = local read "Live Image"() -> (w104:T1)
          }
          frame True {
            n230 = local read "LiveImageBuffer"() -> (w106:T1)
            n231 = local read "IMAQ Session"() -> (w107:T2)
            n232 = call <vilib>:"IMAQdx Grab2.vi"("Image In"=w106, "Session In"=w107) -> ("error out"=w109:errorcluster, "Image Out"=w108:T1)  [unwired: 6 in, 2 out]
            "Live Image" <- w108
          }
        }
        n233 = case shown="True" "AutoPlot" {
          tunnel: w90 -> [_ _]
          tunnel: w89 -> [_ w103]
          tunnel: [_ w94] -> _
          frame False {
          }
          frame True {
            w96 = T8 7 items=["Grayscale (U8)", "Grayscale (I16)", "Grayscale (SGL)", "Complex (CSG)", "RGB (U32)", "HSL (U32)", "RGB (U64)", "Grayscale (U16)"] ("Image Type")
            n234 = call "IMAQ Cast Image"("Image Type"=w96, "Image Src"=w103) -> ("error out"=w95:errorcluster, "Image Dst Out"=w97:T1)  [unwired: 8 in]
            n235 = call "IMAQ ImageToArray"("error in (no error)"=w95, "Image"=w97) -> ("Image Pixels (U16)"=w100:u16[][], "error out"=w94:errorcluster)  [unwired: 2 in, 3 out]
            n236 = call "Eagle Find Spot Pixel.vi"("Image"=w97) -> ("Y Pixel"=w101:i32, "X Pixel"=w102:i32)  [unwired: 8 in, 1 out]
            n237 = Index Array(array=w100, index (col)=w102) -> (element=→"Y Graph":u16[])  [unwired: 1 in]
            n238 = Index Array(array=w100, index (row)=w101) -> (element=→"X Graph":u16[])  [unwired: 1 in]
          }
        }
        n239 = local read "Stopped"() -> (w93:bool)
      }
      n240 = while {
        tunnel: w88 -> [w121]
        stop <- w122 stop-if-true
        n241 = xnode "Read/Write Control"("FPGA VI Reference In"=w121) -> ("X CMD IND"=→"X Command":fxp<+/-,20,5>, "Y CMD IND"=→"Y Command":fxp<+/-,20,5>, "X READ"=→"X Readback" →"X Readback Man":fxp<+/-,20,5>, "Y READ"=→"Y Readback" →"Y Readback Man":fxp<+/-,20,5>, "Manual X IND"=→"X IND":fxp<+/-,20,5>, "Manual Y IND"=→"Y IND":fxp<+/-,20,5>, "Tmp Sens 1"=w113:fxp<+,18,3>, "Tmp Sens 2"=w112:fxp<+,18,3>)  [unwired: 1 in, 2 out]
        n242 = Wait (ms)(milliseconds to wait=u32 100) -> ()  [unwired: 1 out]
        n243 = call "EAGLE Convert Voltage to Temperature.vi"("Tmp Raw 2"=w112, "Tmp Raw 1"=w113) -> ("Temp 2"=→"Sensor 2":dbl, "Temp 1"=→"Sensor 1":dbl)  [unwired: 8 in]
        n244 = local read "Stopped"() -> (w122:bool)
      }
    }
    frame #3 {
      n245 = local read "Images Root Folder"() -> (w369:path)
      n246 = local read "Number Of Points AC"() -> (w376:u16)
      n247 = local read "Dwell Time"() -> (w375:dbl)
      n248 = local read "VX OFFS [Volt] AC"() -> (w374:fxp<+/-,20,5>)
      n249 = local read "VY OFFS [Volt] AC"() -> (w373:fxp<+/-,20,5>)
      n250 = local read "Radius A AC"() -> (w372:dbl)
      n251 = local read "Radius B AC"() -> (w371:dbl)
      n252 = local read "LED Ctrl"() -> (w392:dbl)
      n253 = local read "Red Dots Ctrl"() -> (w391:dbl)
      n254 = local read "Scanner X"() -> (w390:dbl)
      n255 = local read "Scanner Y"() -> (w389:dbl)
      n256 = local read "Radius A"() -> (w388:dbl)
      n257 = local read "Radius B"() -> (w387:dbl)
      n258 = local read "VX OFFS [Volt]"() -> (w377:fxp<+/-,20,5>)
      n259 = local read "VY OFFS [Volt]"() -> (w378:fxp<+/-,20,5>)
      n260 = local read "Number Of Points"() -> (w386:u16)
      n261 = local read "Velocity"() -> (w385:dbl)
      n262 = local read "Tab Control"() -> (w384:T3)
      n263 = Bundle By Name(cluster=T5 {"LedRing_Ctrl"=0.0, "RedDots_Ctrl"=0.0, "VRange_Ctrl"=0.0, "HRange_Ctrl"=0.0, "Aim_Ctrl"=0.0, "ScanX"=0.0, "ScanY"=0.0, "Trajectory"={"Radius A"=0.0, "Radius B"=0.0, "VX OFFS"=0.0, "VY OFFS"=0.0}, "General"={"NumOfPoints"=0, "Velocity"=0.0}, "Tab"=0, "Automatic"={"NumOfPoints"=0, "Dwell Time"=0.0, "VY OFFS"=0.0, "VX OFFS"=0.0, "Radius A"=0.0, "Radius B"=0.0}, "Images Folder"=path ""} ("PanelData"), "LedRing_Ctrl"=w392, "RedDots_Ctrl"=w391, "ScanX"=w390, "ScanY"=w389, "Trajectory.Radius A"=w388, "Trajectory.Radius B"=w387, "Trajectory.VX OFFS"=w377, "Trajectory.VY OFFS"=w378, "General.NumOfPoints"=w386, "General.Velocity"=w385, "Tab"=w384, "Automatic.NumOfPoints"=w376, "Automatic.Dwell Time"=w375, "Automatic.VY OFFS"=w374, "Automatic.VX OFFS"=w373, "Automatic.Radius A"=w372, "Automatic.Radius B"=w371, "Images Folder"=w369) -> (w383:T5)
      n264 = disable-structure shown="RUN_TIME_ENGINE==True" {
        frame condition #0 {
          n265 = Quit LabVIEW(quit? (T)=TRUE) -> ()
        }
        frame condition #1 (active) {
        }
      }
      n266 = local read "IMAQ Session"() -> (w368:T2)
      n267 = Flatten To String(anything=w383) -> (data string=w382:string)  [unwired: 3 in, 2 out]
      n268 = call <vilib>:"Application Directory.vi"() -> ("Application Directory"=w381:path)
      n269 = Build Path(base path=w381, name or relative path="BasicApp_Data.dat") -> (appended path=w379:path)
      n270 = call <vilib>:"IMAQdx Close Camera.vi"("Session In"=w368) -> ()  [unwired: 10 in, 1 out]
      n271 = Write to Text File(file (use dialog)=w379, text=w382) -> ()  [unwired: 2 in, 3 out]
    }
  }
